vi "Inverse3DOFChair.vi"(8 "L 2":dbl(slide)=80.0 scale=0.0..200.0, 9 "L 1":dbl(slide)=80.0 scale=0.0..200.0, 11 "end effector":cluster{dbl, dbl}={80.0, 80.0} {"?" format="%.1f"; "?" format="%#.1f"}) -> (0 "theta2":dbl(knob)=90.0 scale=-90.0..90.0, 1 "theta1":dbl(knob)=-6.3611093629270335e-15 scale=-90.0..90.0, 2 "theta3":dbl(knob)=-90.0 scale=-90.0..90.0)   [LabVIEW 2024]
panel:
  out "L3":dbl=113.13708498984761
  # "mm"
  # "mm"
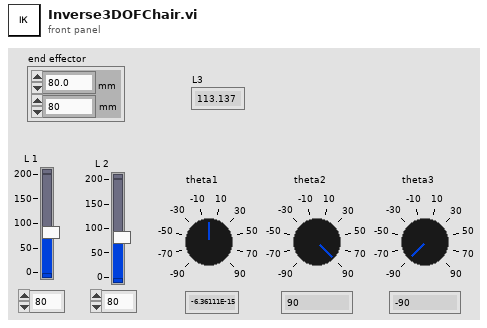
[diagram p1: front panel]
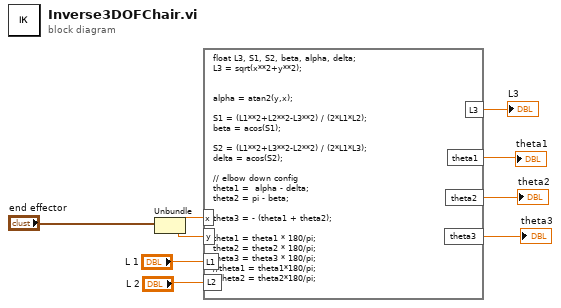
[diagram p0: block diagram]
diagram:
  n1 = Unbundle("end effector") -> (w8:dbl, w7:dbl)
  n2 = formula code="float L3, S1, S2, beta, alpha, delta;\nL3 = sqrt(x**2+y**2);\n\n\nalpha = atan2(y,x);\n\nS1 = (L1**2+L2**2-L3**2) / (2*L1*L2);\nbeta = acos(S1);\n\nS2 = (L1**2+L3**2-L2**2) / (2*L1*L3);\ndelta = acos(S2);\n\n// elbow down config\ntheta1 =  alpha - delta; \ntheta2 = pi - beta;\n\ntheta3 = - (theta1 + theta2);\n\ntheta1 = theta1 * 180/pi;\ntheta2 = theta2 * 180/pi;\ntheta3 = theta3 * 180/pi;\n//theta1 = theta1*180/pi;\n//theta2 = theta2*180/pi;"("L1"="L 1", "L2"="L 2", "x"=w8, "y"=w7) -> ("theta1"=→"theta1":dbl, "theta2"=→"theta2":dbl, "L3"=→"L3":dbl, "theta3"=→"theta3":dbl)
